vi "LEP_RV_UVAddFiles.vi"(0 "uVision Project":path, 1 "Target":string, 2 "VI Group Name":string="VIs", 3 "LV Runtime Group Name":string="Runtime", 4 "Driver Group Name":string="Runtime", 5 "error in (no error)":errorcluster) -> (19 "error out":errorcluster)   [LabVIEW 2011]
doc: "Runs the embedded application on a console located in the <B>Build Path</B> directory ."
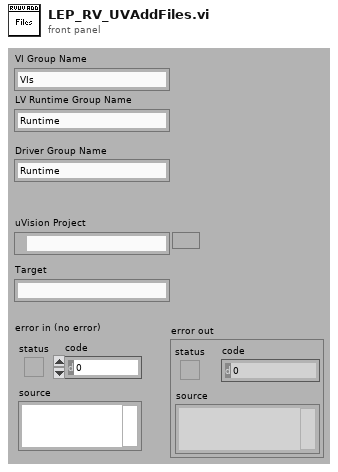
[diagram p1: front panel]
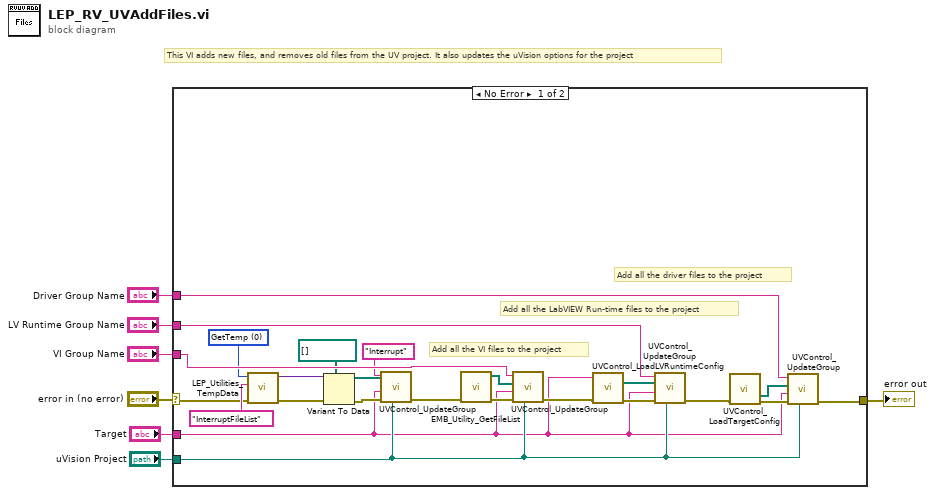
[diagram p0: block diagram]
diagram:
  # "This VI adds new files, and removes old files from the UV project. It also updates the uVision options for the project"
  n1 = case shown="No Error" "error in (no error)" {
    selector: "error in (no error)" -> [w18 w32]
    tunnel: [w17 w32] -> w6
    tunnel: "Target" -> [w9 _]
    tunnel: "VI Group Name" -> [w29 _]
    tunnel: "LV Runtime Group Name" -> [w28 _]
    tunnel: "uVision Project" -> [w16 _]
    tunnel: "Driver Group Name" -> [w15 _]
    frame No Error {
      w22 = u16 0 items=["GetTemp", "SetTemp", "ClearTemp"] ("Command")
      # "Add all the driver files to the project"
      # "Add all the VI files to the project"
      # "Add all the LabVIEW Run-time files to the project"
      n2 = call <vilib>:"LEP_Utilities_TempData.vi"("error in"=w18, "Name"="InterruptFileList", "Command"=w22) -> ("error out"=w25:errorcluster, "Variant Out"=w26:variant)  [unwired: 6 in, 1 out]
      n3 = Variant To Data(error in=w25, type=path[] [], Variant=w26) -> (data=w21:path[], error out=w24:errorcluster)
      n4 = call "UVControl_UpdateGroup.vi"("uVision Project"=w16, "error in (no error)"=w24, "Target"=w9, "Files"=w21, "Group"="Interrupt") -> ("error out"=w19:errorcluster)  [unwired: 6 in]
      n5 = call <vilib>:"EMB_Utility_GetFileList.vi"("error in (no error)"=w19) -> ("error out"=w31:errorcluster, "File List"=w30:path[])  [unwired: 9 in]
      n6 = call "UVControl_UpdateGroup.vi"("uVision Project"=w16, "error in (no error)"=w31, "Target"=w9, "Files"=w30, "Group"=w29) -> ("error out"=w11:errorcluster)  [unwired: 6 in]
      n7 = call "UVControl_LoadLVRuntimeConfig.vi"("Target"=w9, "error in (no error)"=w11) -> ("RunTime C Files"=w8:path[], "error out"=w10:errorcluster)  [unwired: 8 in, 4 out]
      n8 = call "UVControl_UpdateGroup.vi"("uVision Project"=w16, "error in (no error)"=w10, "Target"=w9, "Files"=w8, "Group"=w28) -> ("error out"=w14:errorcluster)  [unwired: 6 in]
      n9 = call "UVControl_LoadTargetConfig.vi"("error in (no error)"=w14) -> ("Driver C Files"=w12:path[], "error out"=w13:errorcluster)  [unwired: 9 in, 4 out]
      n10 = call "UVControl_UpdateGroup.vi"("uVision Project"=w16, "error in (no error)"=w13, "Target"=w9, "Files"=w12, "Group"=w15) -> ("error out"=w17:errorcluster)  [unwired: 6 in]
    }
    frame Error {
    }
  }
  "error out" <- w6
